vi "write_lv_signal.vi"(4 "Small?":bool, 7 "Index":i32, 8 "error in":errorcluster, 9 "File Name":string="\\", 10 "Save Path":path, 11 "Signal array":T1[](array[typedef])) -> (0 "error out":errorcluster)   [LabVIEW 2013]
uses:
  Public API/Signal.ctl
  Role ID.ctl
  Hardware ID.ctl
  Batch Processor/bp_cluster.ctl
  File_location.ctl
panel:
  out "concatenated string":string
  # "Signal"
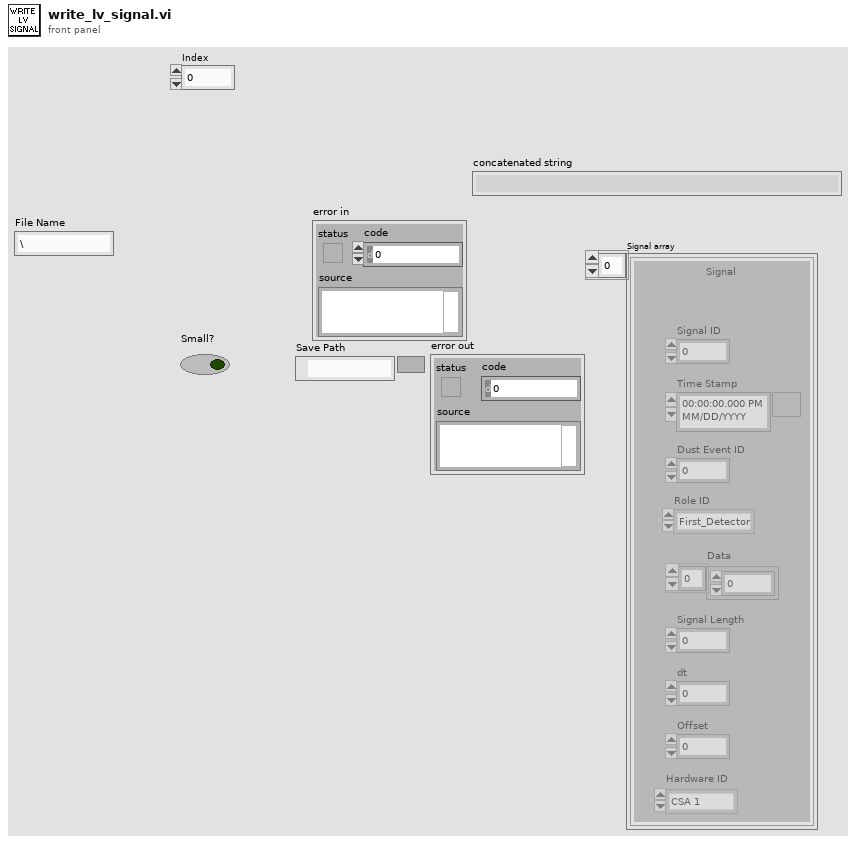
[diagram p1: front panel]
types:
  T1 = typedef "Signal.ctl" = cluster{"Signal ID":i64, "Time Stamp":timestamp, "Dust Event ID":i64, "Role ID":T2, "Data":sgl[], "Signal Length":i32, "dt":sgl, "Offset":dbl, "Hardware ID":T3}
  T2 = typedef "Role ID.ctl" = enum16{"First_Detector", "Second_Detector", "Third_Detector", "LeCroy_CH1", "LeCroy_CH2", "LeCroy_CH3", "LeCroy_CH4", "PSU"}
  T3 = typedef "Hardware ID.ctl" = enum16{"Unknown", "CSA 1", "CSA 2", "CSA 3", "CSA 4", "CSA 5", "CSA 6"}
  T4 = typedef "bp_cluster.ctl" = cluster{"Dust Event ID":i64, "High Voltage":sgl, "Experiment Settings  ID":i64, "File Location":T5, "Dust Density":dbl}
  T5 = typedef "File_location.ctl" = i8
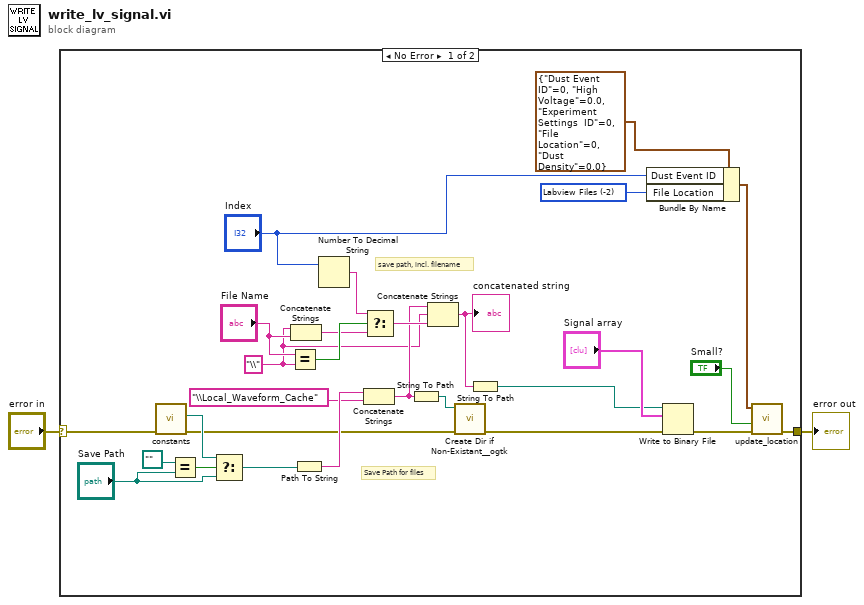
[diagram p0: block diagram]
diagram:
  n1 = case shown="No Error" "error in" {
    selector: "error in" -> [w29 w31]
    tunnel: [w12 w31] -> w1
    frame No Error {
      w10 = T5 -2 items=["Labview Files"=-2, "Mars Data Processing Factility"=-1, "Local Cache "=0, "Old Storage"=1, "Storage"=2] ("File Location")
      w3 = "\\" ("y")
      # "save path, incl. filename"
      # "Save Path for files"
      n2 = call "constants.vi"("error in (no error)"=w29) -> ("error out"=w8:errorcluster, "file path for Signal .hdf5 files"=w26:path)  [unwired: 4 in, 5 out]
      n3 = Equal?(x=path "" ("Save Path"), y="Save Path") -> (x = y?=w25:bool)
      n4 = Select(t=w26, s=w25, f="Save Path") -> (s? t:f=w28:path)
      n5 = Equal?(x="File Name", y=w3) -> (x = y?=w23:bool)
      n6 = Concatenate Strings(w3, "File Name") -> (w22:string)
      n7 = Path To String(path=w28) -> (string=w18:string)
      n8 = Number To Decimal String(number="Index") -> (decimal integer string=w20:string)  [unwired: 1 in]
      n9 = Concatenate Strings(w18, "\\Local_Waveform_Cache" ("string")) -> (w17:string)
      n10 = Select(t=w20, s=w23, f=w22) -> (s? t:f=w19:string)
      n11 = String To Path(string=w17) -> (path=w6:path)
      n12 = Concatenate Strings(w17, w3, w19) -> (w30:string)
      "concatenated string" <- w30
      n13 = call <userlib>:"Create Dir if Non-Existant__ogtk.vi"("error in (no error)"=w8, "Directory Path"=w6) -> ("error out"=w7:errorcluster)  [unwired: 7 in, 2 out]
      n14 = String To Path(string=w30) -> (path=w5:path)
      n15 = Bundle By Name(cluster=T4 {"Dust Event ID"=0, "High Voltage"=0.0, "Experiment Settings  ID"=0, "File Location"=0, "Dust Density"=0.0} ("Batch Processing Cluster"), "Dust Event ID"="Index", "File Location"=w10) -> (w14:T4)
      n16 = Write to Binary File(file (use dialog)=w5, data="Signal array", error in=w7) -> (error out=w13:errorcluster)  [unwired: 3 in, 2 out]
      n17 = call "update_location.vi"("error in (no error)"=w13, "Small?"="Small?", "Batch Processing Cluster"=w14) -> ("error out"=w12:errorcluster)  [unwired: 7 in, 1 out]
    }
    frame Error {
    }
  }
  "error out" <- w1
